vi "Bearer Token.vi"(8 "error in (no error)":errorcluster, 11 "Gmail in":refnum<class "Gmail.lvclass">) -> (0 "error out":errorcluster, 2 "Bearer Token":string, 3 "Gmail out":refnum<class "Gmail.lvclass">)   [LabVIEW 2020, in "Gmail API.lvlib" / "Gmail.lvclass"]
uses:
  Gmail.lvclass
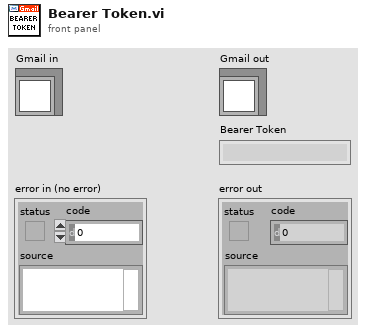
[diagram p1: front panel]
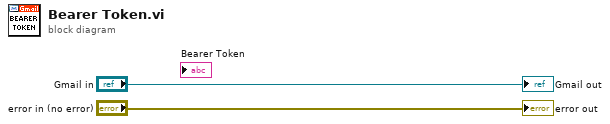
[diagram p0: block diagram]
diagram:
  "error out" <- "error in (no error)"
  "Gmail out" <- "Gmail in"
